vi "ma_Get Waveform Info (CDB).vi"(11 "time signal in":waveform(cdb)) -> (0 "spectral info":T1 {"window" items=["Rectangle"=0, "Hanning"=1, "Hamming"=2, "Blackman-Harris"=3, "Exact Blackman"=4, "Blackman"=5, "Flat Top"=6, "4 Term B-Harris "=7, "7 Term B-Harris"=8, "Low Sidelobe"=9, "Blackman Nuttall"=11, "Triangle"=30, "Bartlett-Hanning"=31, "Bohman"=32, "Parzen"=33, "Welch"=34, "Kaiser"=60, "Dolph-Chebyshev"=61, "Gaussian"=62]}, 1 "df":dbl, 2 "fs":dbl, 3 "f0":dbl)   [LabVIEW 2020, in "NI_MAPro.lvlib"]
uses:
  NI_MAPro.lvlib
  ma_sml_Spectral Info.ctl
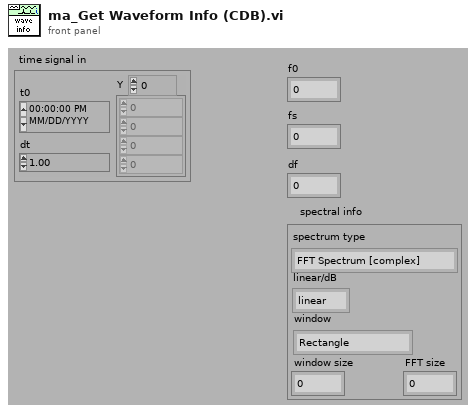
[diagram p1: front panel]
types:
  T1 = typedef "NI_MAPro.lvlib/ma_sml_Spectral Info.ctl" = cluster{"spectrum type":enum16{"FFT Spectrum [complex]", "Amplitude [Magnitude]", "Power [Magnitude^2]", "Cross Spectrum [complex]", "Frequency Response [Complex]"}, "linear/dB":enum16{"linear", "dB"}, "window":u16, "window size":i32, "FFT size":i32}
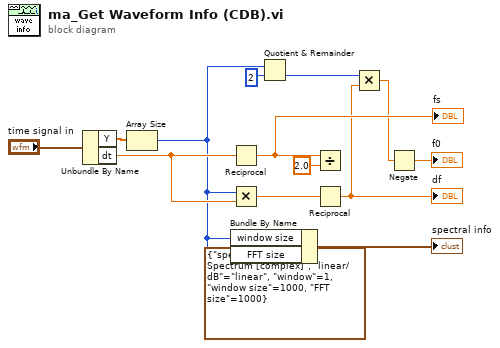
[diagram p0: block diagram]
diagram:
  n1 = Unbundle By Name("time signal in") -> ("Y"=w14:cdb[], "dt"=w9:dbl)
  n2 = Array Size(array=w14) -> (size(s)=w4:i32)
  n3 = Reciprocal(x=w9) -> (1/x=w6:dbl)
  "fs" <- w6
  n4 = Multiply(x=w4, y=w9) -> (x*y=w10:dbl)
  n5 = Bundle By Name(cluster=T1 {"spectrum type"=enum."FFT Spectrum [complex]", "linear/dB"=enum."linear", "window"=1, "window size"=1000, "FFT size"=1000} ("spectral info"), "window size"=w4, "FFT size"=w4) -> (→"spectral info":T1)
  n6 = Quotient & Remainder(x=w4, y=2) -> (floor(x/y)=w3:i32)  [unwired: 1 out]
  n7 = Divide(x=w6, y=2.0) -> ()  [unwired: 1 out]
  n8 = Reciprocal(x=w10) -> (1/x=w2:dbl)
  "df" <- w2
  n9 = Multiply(x=w3, y=w2) -> (x*y=w1:dbl)
  n10 = Negate(x=w1) -> (-x=→"f0":dbl)
